vi "Flowrate.vi"() -> ()   [LabVIEW 2018, in "com.Instrument.lvlib"]
uses:
  com.Instrument.lvlib
  <vilib>/measure/NI_MAPro.lvlib
  <vilib>/measure/mascope.llb/Pulse Measurements 1 chan.vi
panel:
  out "period":dbl format="%.2g"
  in  "signal in":waveform(dbl)={"t0"=timestamp(0 s since 1904-01-01), "dt"=0.0, "Y"=[]}
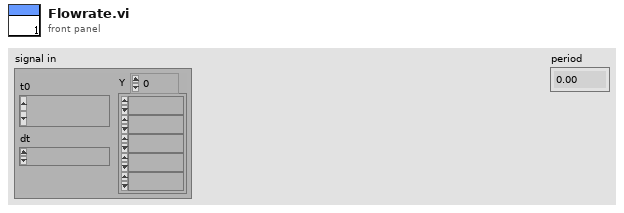
[diagram p1: front panel]
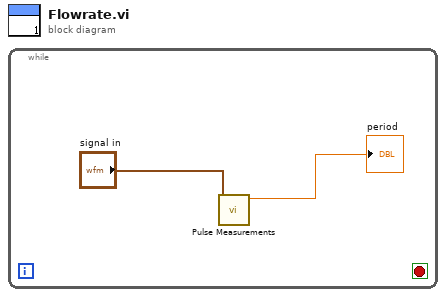
[diagram p0: block diagram]
diagram:
  n1 = while {
    stop <- _ stop-if-true
    n2 = call-poly <vilib>:"Pulse Measurements.vi"("signal in"="signal in") -> ("period"=→"period":dbl)  [unwired: 6 in, 4 out]
  }
